vi "Gui_SetupTrapping.vi"(8 "error in (no error)":errorcluster, 10 "Variant for Path":variant, 11 "Variant":variant) -> (0 "error out":errorcluster caption="sortie d'erreur", 3 "Variant out":variant)   [LabVIEW 2018]
uses:
  controls/SEQUENCE_Inputs.ctl
  controls/EXCIT_Inputs.ctl
  controls/DATA_Inputs.ctl
  controls/TIMING_Inputs.ctl
  controls/PROCESSING_Inputs.ctl
  controls/TRAPPING_Inputs.ctl
  controls/EXPERT_Inputs.ctl
  controls/DIGIT_5122_Inputs.ctl
  <instrlib>/niScope/Controls/niScope trigger source.ctl
  controls/HSDIO_6541_Inputs.ctl
  <instrlib>/niHSDIO/niHSDIO.llb/niHSDIO_ctl Trigger Source Values (Ring).ctl
  controls/SOFTWARE_Inputs.ctl
  controls/AO_6711_Inputs.ctl
  controls/AWG_5421_Inputs.ctl
  <instrlib>/niFgen/niFgen.llb/niFgen_ctl Trigger Source Values (Ring).ctl
  controls/XML_Inputs.ctl
panel:
  in  "TRAPPING Inputs":T1={"Number of Channels"=4, "Init Values"=[2.0, 9.0, 2.0, 9.0], "Opening Values"=[0.0, 0.0, 0.0, 0.0], "Trapping Values"=[2.0, 9.0, 2.0, 9.0], "Emptying Values"=[-10.0, -10.0, -10.0, -10.0], "Adiabatic ON"=FALSE, "Adiabatic Duration"=100, "Adiabatic Waveforms"=["Adiabatic_None_2_2_2000", "Adiabatic_Ramp_9_0_2000", "Adiabatic_None_2_2_2000", "Adiabatic_RC_9_0_2000"], "Ions Refill ON"=FALSE, "Number of Ions Refills"=1, "Trapping Delay"=400.0, "Trapping Duration"=300.0} {"Trapping Duration" min=2.0; "Trapping Delay" min=2.0; "Number of Ions Refills" min=1 max=1000; "Trapping Values" min=-10.0 max=10.0; "Init Values" min=-10.0 max=10.0; "Emptying Values" min=-10.0 max=10.0; "Opening Values" min=-10.0 max=10.0}
  in  "SEQUENCE Inputs":T2={"EXCIT Inputs"={"Number of Excitations"=1, "Script Text"="", "Table of Waveforms"=[]}, "DATA Inputs"={"Record Length"=8192, "Sample Rate"=4.0, "Data Type"=0, "Vertical Range"=0.0, "Acquisition Duration"=100000.0}, "TIMING Inputs"={"Number of Acquisitions "=1, "Number of Accumulations"=1, "Table of Waveforms"=[], "Script Text"=""}, "PROCESSING Inputs"={"Reference Mass"=300.0939, "Cyclotron Freq"=255.727, "Magnetron Freq"=0.001}, "TRAPPING Inputs"={"Number of Channels"=4, "Init Values"=[2.0, 5.0, 5.0, 2.0], "Opening Values"=[0.0, 0.0, 0.0, 0.0], "Trapping Values"=[2.0, 5.0, 5.0, 2.0], "Emptying Values"=[-5.0, -5.0, -5.0, -5.0], "Adiabatic ON"=FALSE, "Adiabatic Duration"=0, "Adiabatic Waveforms"=["Adiabatic_None_2_2_2000.bin", "Adiabatic_Ramp_5_0_2000.bin", "Adiabatic_DoubleRamp_5_0_2000.bin", "Adiabatic_RC_2_0_2000.bin"], "Ions Refill ON"=FALSE, "Number of Ions Refills"=4, "Trapping Delay"=400.0, "Trapping Duration"=300.0}} {"TRAPPING Inputs"."Trapping Duration" min=2.0; "TRAPPING Inputs"."Trapping Delay" min=2.0; "TRAPPING Inputs"."Number of Ions Refills" min=1 max=1000; "TRAPPING Inputs"."Trapping Values" min=-10.0 max=10.0; "TRAPPING Inputs"."Init Values" min=-10.0 max=10.0; "TRAPPING Inputs"."Emptying Values" min=-10.0 max=10.0; "TRAPPING Inputs"."Opening Values" min=-10.0 max=10.0; "PROCESSING Inputs"."Magnetron Freq" format="%.5g"; "PROCESSING Inputs"."Cyclotron Freq" format="%.5g"; "PROCESSING Inputs"."Reference Mass" format="%.5g"; "TIMING Inputs"."Number of Accumulations" min=0 max=50 step=1; "TIMING Inputs"."Number of Acquisitions" min=1 max=10 step=1; "DATA Inputs"."Vertical Range" items=["0.2"=0.2, "0.4"=0.4, "1"=1.0, "2"=2.0, "4"=4.0, "10"=10.0]; "DATA Inputs"."Data Type" items=["I16", "DBL"]; "DATA Inputs"."Sample Rate" items=["1 MHz"=1000000.0, "2 MHz"=2000000.0, "5 MHz"=5000000.0, "10 MHz"=10000000.0, "20 MHz"=20000000.0, "25 MHz"=25000000.0, "50 MHz"=50000000.0, "100 MHz"=100000000.0]; "EXCIT Inputs"."Number of Excitations" min=1 max=10}
  in  "OK":bool
  # "GO_out"
  # "Gout"
  # "GI_in"
  # "Gin"
  # "GO_out"
  # "Gout"
  # "GI_in"
  # "Gin"
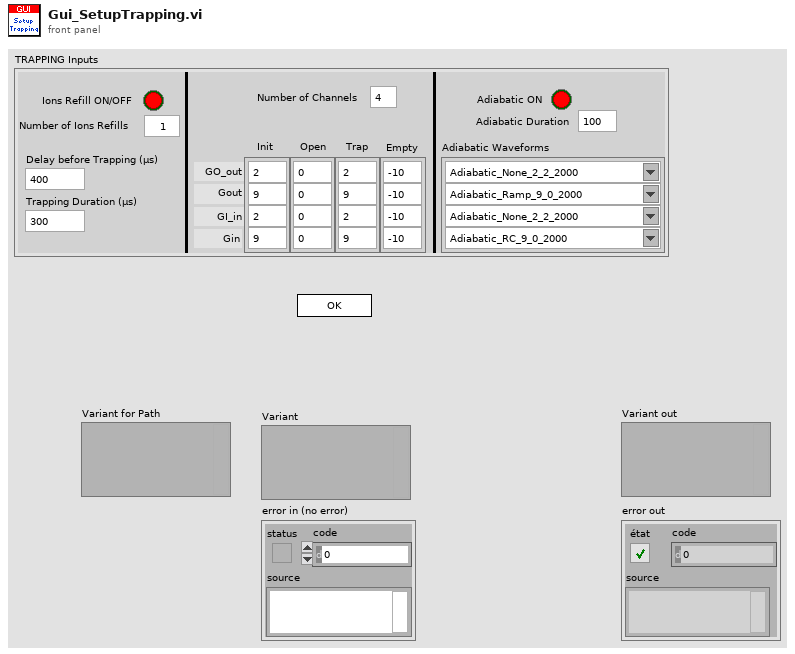
[diagram p1: front panel]
types:
  T1 = typedef "TRAPPING_Inputs.ctl" = cluster{"Number of Channels":i32, "Init Values":dbl[], "Opening Values":dbl[], "Trapping Values":dbl[], "Emptying Values":dbl[], "Adiabatic ON":bool, "Adiabatic Duration":i32, "Adiabatic Waveforms":string[], "Ions Refill ON":bool, "Number of Ions Refills":i32, "Trapping Delay":dbl, "Trapping Duration":dbl}
  T2 = typedef "SEQUENCE_Inputs.ctl" = cluster{"EXCIT Inputs":T3, "DATA Inputs":T4, "TIMING Inputs":T5, "PROCESSING Inputs":T6, "TRAPPING Inputs":T1}
  T3 = typedef "EXCIT_Inputs.ctl" = cluster{"Number of Excitations":i32, "Script Text":string, "Table of Waveforms":string[]}
  T4 = typedef "DATA_Inputs.ctl" = cluster{"Record Length":i32, "Sample Rate":dbl, "Data Type":u8, "Vertical Range":dbl, "Acquisition Duration":dbl}
  T5 = typedef "TIMING_Inputs.ctl" = cluster{"Number of Acquisitions ":i16, "Number of Accumulations":i16, "Table of Waveforms":string[], "Script Text":string}
  T6 = typedef "PROCESSING_Inputs.ctl" = cluster{"Reference Mass":dbl, "Cyclotron Freq":dbl, "Magnetron Freq":dbl}
  T7 = typedef "EXPERT_Inputs.ctl" = cluster{"DIGIT 5122 Inputs":T8, "HSDIO 6541 Inputs":T10, "SOFTWARE Inputs":T12, "AO 6711 Inputs":T13, "AWG 5421 Inputs":T14, "XML Inputs":T16}
  T8 = typedef "DIGIT_5122_Inputs.ctl" = cluster{"Sample Rate":dbl, "Resource Name":refnum<k15>, "Channel Name":string, "Trigger Source":T9, "Vertical Range":dbl, "Trigger Level":dbl}
  T9 = typedef "niScope trigger source.ctl" = string
  T10 = typedef "HSDIO_6541_Inputs.ctl" = cluster{"Resource Name":refnum<k15>, "Clock Rate":dbl, "Trigger Source":T11}
  T11 = typedef "niHSDIO_ctl Trigger Source Values (Ring).ctl" = string
  T12 = typedef "SOFTWARE_Inputs.ctl" = cluster{"Application Directory":path, "Software Version":string, "Data Path":path, "XML Path":path, "XML File Filter":string, "XML Saved Path":path, "Excit Scripts Path":path, "Excit Scripts File Filter":string, "Excit Waveforms Path":path, "Excit Waveforms File Filter":string, "Timing Scripts Path":path, "Timing Scripts File Filter":string, "Timing Waveforms Path":path, "Timing Waveforms File Filter":string, "Trapping Waveforms Path":path, "Trapping Waveforms File Filter":string}
  T13 = typedef "AO_6711_Inputs.ctl" = cluster{"Physical Channels":tag, "Min Voltage":dbl, "Max Voltage":dbl, "Trigger Source":tag, "Counter":tag}
  T14 = typedef "AWG_5421_Inputs.ctl" = cluster{"Resource Name":refnum<k15>, "Sample Rate":dbl, "Trigger Type":u16, "Trigger Source":T15, "Waveform Gain":dbl, "Digital Filter ON":bool}
  T15 = typedef "niFgen_ctl Trigger Source Values (Ring).ctl" = string
  T16 = typedef "XML_Inputs.ctl" = cluster{"Version Tag Name":string, "Version String":string}
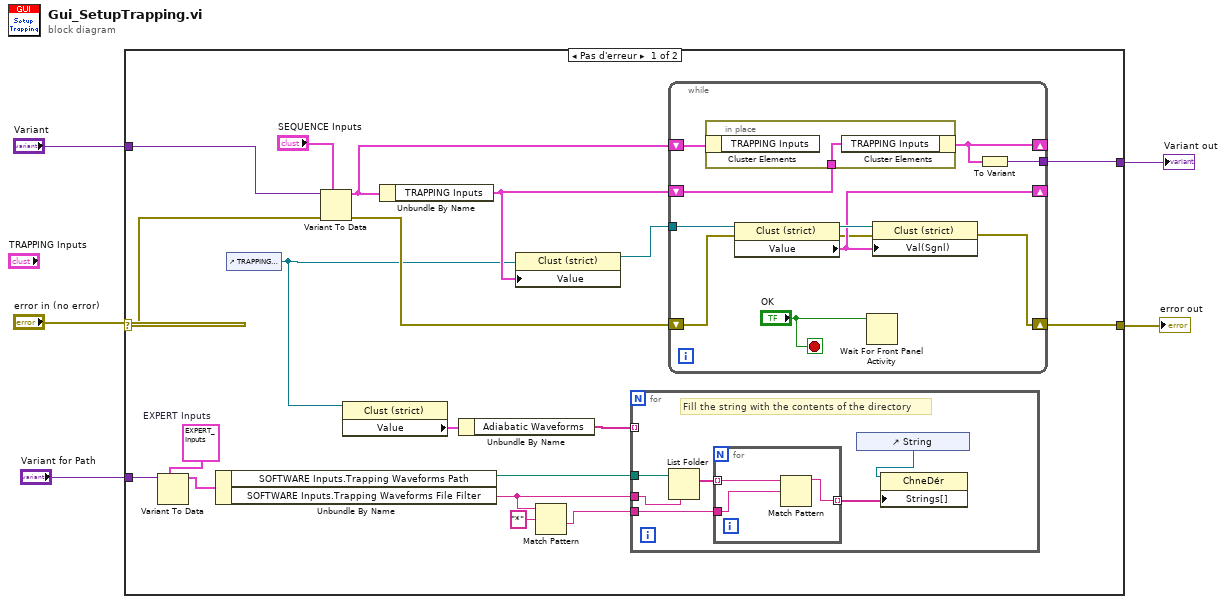
[diagram p0: block diagram]
diagram:
  n1 = case shown="Pas d'erreur" "error in (no error)" {
    selector: "error in (no error)" -> [w20 w47]
    tunnel: [w24 w47] -> w4
    tunnel: "Variant" -> [w22 w46]
    tunnel: [w7 w46] -> w2
    tunnel: "Variant for Path" -> [w16 _]
    frame No Error {
      w15 = T7 {"DIGIT 5122 Inputs"={"Sample Rate"=10000.0, "Resource Name"="DIGIT_5122", "Channel Name"="0", "Trigger Source"="VAL_EXTERNAL", "Vertical Range"=10.0, "Trigger Level"=3.0}, "HSDIO 6541 Inputs"={"Resource Name"="HSDIO_6541", "Clock Rate"=1000000.0, "Trigger Source"="PFI0"}, "SOFTWARE Inputs"={"Application Directory"=path "D:/S.O.F.T.S/LABVIEW/PIL", "Software Version"="1.0.0", "Data Path"=path "D:/PIRENEA/DATA", "XML Path"=path "D:/PIRENEA/DATA", "XML File Filter"="*.xml", "XML Saved Path"=path "D:/PIRENEA/DATA/SAVED", "Excit Scripts Path"=path "D:/PIRENEA/EXCIT_SCRIPTS", "Excit Scripts File Filter"="*.txt", "Excit Waveforms Path"=path "D:/PIRENEA/EXCIT_WFMS", "Excit Waveforms File Filter"="*.bin", "Timing Scripts Path"=path "D:/PIRENEA/TIMING_SCRIPTS", "Timing Scripts File Filter"="*.txt", "Timing Waveforms Path"=path "D:/PIRENEA/TIMING_WFMS", "Timing Waveforms File Filter"="*.bin", "Trapping Waveforms Path"=path "D:/PIRENEA/TRAPPING_WFMS", "Trapping Waveforms File Filter"="*.bin"}, "AO 6711 Inputs"={"Physical Channels"="AO_6711/ao0:3", "Min Voltage"=-10.0, "Max Voltage"=10.0, "Trigger Source"="/AO_6711/PFI3", "Counter"="AO_6711/ctr0"}, "AWG 5421 Inputs"={"Resource Name"="AWG_5421", "Sample Rate"=10000000.0, "Trigger Type"=2, "Trigger Source"="PFI0", "Waveform Gain"=0.31, "Digital Filter ON"=TRUE}, "XML Inputs"={"Version Tag Name"="XML_Version", "Version String"="1.0"}}  # EXPERT Inputs
      n2 = Variant To Data(type=w15, Variant=w16) -> (data=w14:T7)  [unwired: 1 in, 1 out]
      n3 = Unbundle By Name(w14) -> ("SOFTWARE Inputs.Trapping Waveforms Path"=w17:path, "SOFTWARE Inputs.Trapping Waveforms File Filter"=w13:string)
      n4 = control-ref of="TRAPPING Inputs"() -> (w6:refnum<vi>)
      n5 = Variant To Data(error in=w20, type="SEQUENCE Inputs", Variant=w22) -> (data=w21:T2, error out=w19:errorcluster)
      n6 = property class="Clust (strict)"(reference=w6) -> ("Value"=w9:T1)  [unwired: 1 in, 2 out]
      n7 = Unbundle By Name(w21) -> ("TRAPPING Inputs"=w18:T1)
      n8 = Unbundle By Name(w9) -> ("Adiabatic Waveforms"=w8:string[])
      n9 = property class="Clust (strict)"(reference=w6, "Value"=w18) -> (reference out=w10:refnum<vi>)  [unwired: 1 in, 1 out]
      n10 = Match Pattern(string=w13, regular expression="*" ("expression régulière")) -> (after substring=w11:string)  [unwired: 1 in, 3 out]
      n11 = for {
        tunnel: w17 -> [w28]
        tunnel: w13 -> [w27]
        tunnel: w11 -> [w26]
        tunnel: w8 -> [_] mode=indexing
        # "Fill the string with the contents of the directory"
        n12 = List Folder(path=w28, pattern=w27) -> (filenames=w30:string[])  [unwired: 2 in, 3 out]
        n13 = for {
          tunnel: w30 -> [w33] mode=indexing
          tunnel: [w32] -> w29 mode=indexing
          tunnel: w26 -> [w31]
          n14 = Match Pattern(string=w33, regular expression=w31) -> (before substring=w32:string)  [unwired: 1 in, 3 out]
        }
        n15 = control-ref of="String"() -> (w25:refnum<vi>)
        n16 = property class="ChneDér"(reference=w25, "Strings[]"=w29) -> ()  [unwired: 1 in, 2 out]
      }
      n17 = while {
        shift-right: [w38] -> w24
        shift-left: w19 -> [w40]
        shift-right: [w34] -> _
        shift-left: w21 -> [w44]
        shift-right: [w42] -> _
        shift-left: w18 -> [w41]
        tunnel: w10 -> [w36]
        tunnel: [w35] -> w7
        stop <- "OK" stop-if-true
        n18 = in-place {
          in-place-border: w41 -> [w45]
          n19 = in-place-cluster #1(w44) -> ()  [unwired: 1 out]
          n20 = in-place-cluster #1("TRAPPING Inputs"=w45) -> (w34:T2)
        }
        n21 = property class="Clust (strict)"(reference=w36, error in=w40) -> (reference out=w43:refnum<vi>, error out=w39:errorcluster, "Value"=w42:T1)
        n22 = Wait For Front Panel Activity(3:"OK") -> ()  [unwired: 2 in, 1 out]
        n23 = property class="Clust (strict)"(reference=w43, error in=w39, "Val(Sgnl)"=w42) -> (error out=w38:errorcluster)  [unwired: 1 out]
        n24 = To Variant(anything=w34) -> (Variant=w35:variant)
      }
    }
    frame Error {
    }
  }
  "error out" <- w4
  "Variant out" <- w2
